vi "sv_Assign Delay to Idle Channels_Copy.vi"(7 "tolerance":dbl=0.1 format="%#_13g", 9 "delays [s] in":dbl[](array[numeric]), 10 "coherences":dbl[](array[numeric]), 11 "acquired responses":waveform(dbl)[](array[waveform])) -> (1 "delays [s] out":dbl[](array[numeric]), 2 "verified":bool, 3 "acquired responses dup":waveform(dbl)[](array[waveform]))   [LabVIEW 2021, in "Audio ADC Shared.lvlib"]
doc: "To assign a delay for each idle channel in which the sync pulse coherence is below threshold, this VI finds a channel with same units and coherence greater than threshold and assigns that delay to idle channel."
uses:
  <vilib>/addons/_NISVFA/_Shared subVIs/Controls/NI Channel Properties.ctl
  Audio ADC Shared.lvlib
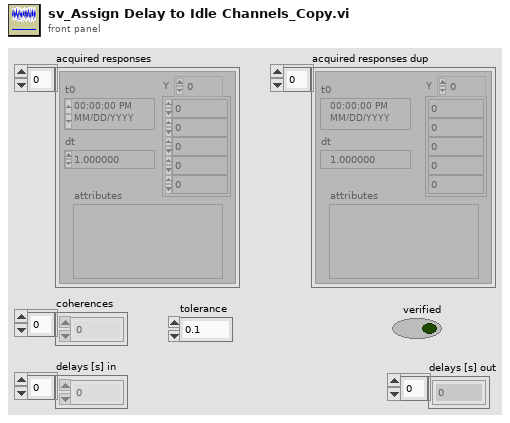
[diagram p1: front panel]
types:
  T1 = typedef "NI Channel Properties.ctl" = u16
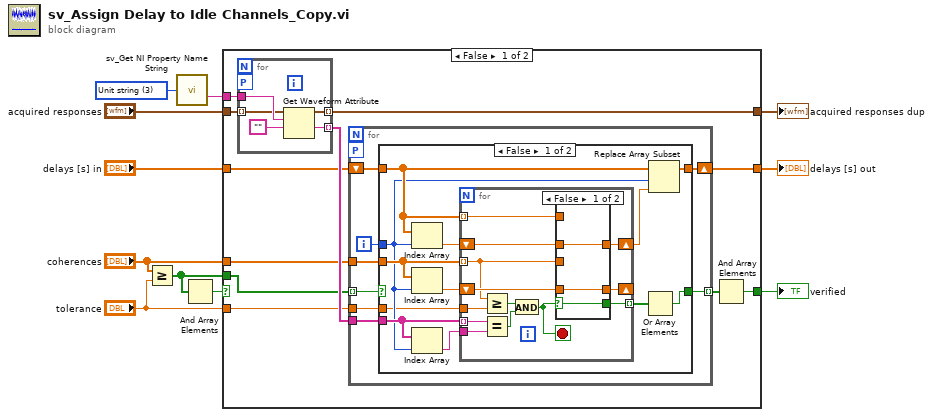
[diagram p0: block diagram]
diagram:
  w9 = T1 3 items=["Channel name", "Channel description", "Axis label", "Unit string", "Waveform X-axis label", "Waveform X-axis unit string", "x0", "dx", "Number of samples", "X channel", "Filter settled", "dB reference", "Window", "Window parameter", "Window size", "FFT size", "Peak units", "Spectrum type", "Magnitude scale", "Spectral density", "Sensor sensitivity (mV/EU)", "X-axis dimension", "LabVIEW datatype", "Function type", "Function subtype", "X values", "Independent channel", "Column index", "Collection name", "Collection ID", "X Columns", "Phase unwrapped", "Sensor type", "Sensor maximum", "Averaging mode"] ("property")
  n1 = Greater Or Equal?(x="coherences", y="tolerance") -> (x >= y?=w1:bool[])
  n2 = call <vilib>:"sv_Get NI Property Name String.vi"("property"=w9) -> ("WDT attribute name"=w10:string)  [unwired: 13 in, 1 out]
  n3 = And Array Elements(Boolean array=w1) -> (logical AND=w2:bool)
  n4 = case shown="False" w2 {
    selector: w2 -> [_ w71]
    tunnel: w1 -> [w16 _]
    tunnel: [w19 w71] -> w3
    tunnel: "coherences" -> [w15 _]
    tunnel: "acquired responses" -> [w21 w69]
    tunnel: "delays [s] in" -> [w17 w70]
    tunnel: [w13 w70] -> w7
    tunnel: [w20 w69] -> w8
    tunnel: w10 -> [w22 _]
    tunnel: "tolerance" -> [w14 _]
    frame False {
      n5 = for {
        tunnel: w22 -> [w67]
        tunnel: w21 -> [w66] mode=indexing
        tunnel: [w65] -> w20 mode=indexing
        tunnel: [w64] -> w18 mode=indexing
        workers-P: _ -> [_]
        n6 = Get Waveform Attribute(5:"" ("Empty String Constant"), 6:w67, 7:w66) -> (1:w64:string, 3:w65:waveform(dbl))  [unwired: 1 in, 2 out]
      }
      n7 = for {
        tunnel: w16 -> [w30] mode=indexing
        tunnel: w15 -> [w28]
        tunnel: w18 -> [w26]
        shift-right: [w27] -> w13
        shift-left: w17 -> [w29]
        tunnel: [w24] -> w12 mode=indexing
        tunnel: w14 -> [w23]
        workers-P: _ -> [_]
        i -> [w25]
        n8 = case shown="False" w30 {
          selector: w30 -> [_ w62]
          tunnel: w29 -> [w35 w63]
          tunnel: w28 -> [w37 _]
          tunnel: [w39 w63] -> w27
          tunnel: w26 -> [w42 _]
          tunnel: w25 -> [w32 _]
          tunnel: [w33 w62] -> w24
          tunnel: w23 -> [w31 _]
          frame False {
            n9 = Index Array(array=w35, index=w32) -> (element=w40:dbl)
            n10 = Index Array(array=w37, index=w32) -> (element=w36:dbl)
            n11 = Index Array(array=w42, index=w32) -> (element=w41:string)
            n12 = for {
              tunnel: w42 -> [w55] mode=indexing
              tunnel: w41 -> [w54]
              tunnel: w37 -> [w47] mode=indexing
              shift-right: [w50] -> w38
              shift-left: w40 -> [w49]
              shift-right: [w52] -> _
              shift-left: w36 -> [w51]
              tunnel: w35 -> [w48] mode=indexing
              tunnel: [w44] -> w34 mode=indexing
              tunnel: w31 -> [w46]
              stop <- w43 stop-if-true
              n13 = Greater Or Equal?(x=w47, y=w46) -> (x >= y?=w45:bool)
              n14 = Equal?(x=w55, y=w54) -> (x = y?=w53:bool)
              n15 = And(x=w45, y=w53) -> (x .and. y?=w43:bool)
              n16 = case shown="False" w43 {
                selector: w43 -> [w56 w59]
                tunnel: [w58 w60] -> w52
                tunnel: w51 -> [w58 _]
                tunnel: [w57 w61] -> w50
                tunnel: w49 -> [w57 _]
                tunnel: w47 -> [_ w60]
                tunnel: w48 -> [_ w61]
                tunnel: [w56 w59] -> w44
                frame False {
                }
                frame True {
                }
              }
            }
            n17 = Or Array Elements(Boolean array=w34) -> (logical OR=w33:bool)
            n18 = Replace Array Subset(array=w35, new element=w38, index=w32) -> (w39:dbl[])
          }
          frame True {
          }
        }
      }
      n19 = And Array Elements(Boolean array=w12) -> (logical AND=w19:bool)
    }
    frame True {
    }
  }
  "acquired responses dup" <- w8
  "delays [s] out" <- w7
  "verified" <- w3
